vi "IMAQ FPGA FIFO to Pixel Bus RGB32x1.vi"(6 "Ready For Output":bool=TRUE, 10 "Image Size":T2, 11 "Source Image FIFO":refnum<k21>) -> (0 "Output Valid":bool, 2 "Source FIFO Status":T1, 3 "Pixel Bus Out":T3)   [LabVIEW 2017, in "NI_VDM_FPGA_Basics.lvlib"]
doc: "Reads image pixels out of the specified FIFO and returns a Pixel Bus cluster of the requested type. The Pixel Bus contains the pixel data from the FIFO along with some additional flags that indicate when the pixel data is valid, an end of a line has been reached, or an end of the image has been reached. The Pixel Bus is used to pass image data to all of the other VIs in the NI Vision Development Module for FPGA library. Only one of the DV, EOL, and EOI flags in the Pixel Bus cluster will assert on a given clock cycle. When the last pixel of an image is reached, the Pixel Bus will contain the pixel data and the DV flag will be TRUE and the EOL and EOI flags will be FALSE. The next clock cycle, the EOL flag will be TRUE and the DV and EOI flags will be FALSE. The following clock cycle, the EOI flag will be TRUE and the DV and EOL flags will be FALSE."
uses:
  <vilib>/visionFPGA/NI_VDM_FPGA_Basics.lvlib
  <vilib>/rvi/DataTransferAndStorage/Container/XNode/niFpgaContainer.xnode
  <vilib>/rvi/FIFO/Fifo_Resource/niFpgaFifoEmulationRefIn.vi
  <vilib>/visionFPGA/Controls/IMAQ FPGA Pixel Bus RGB32x1.ctl
  <vilib>/visionFPGA/Controls/IMAQ FPGA Source FIFO Status.ctl
  <vilib>/visionFPGA/Controls/IMAQ FPGA Image Size.ctl
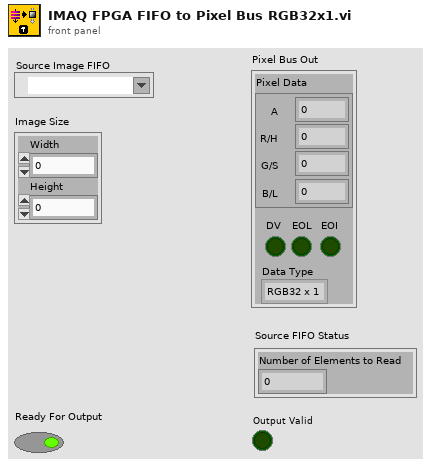
[diagram p1: front panel]
types:
  T1 = typedef "IMAQ FPGA Source FIFO Status.ctl" = cluster{"Number of Elements to Read":u32}
  T2 = typedef "IMAQ FPGA Image Size.ctl" = cluster{"Width":u32, "Height":u32}
  T3 = typedef "IMAQ FPGA Pixel Bus RGB32x1.ctl" = cluster{"Pixel Data":cluster{"A":u8, "R/H":u8, "G/S":u8, "B/L":u8}, "DV":bool, "EOL":bool, "EOI":bool, "Data Type":enum16{"RGB32 x 1"}}
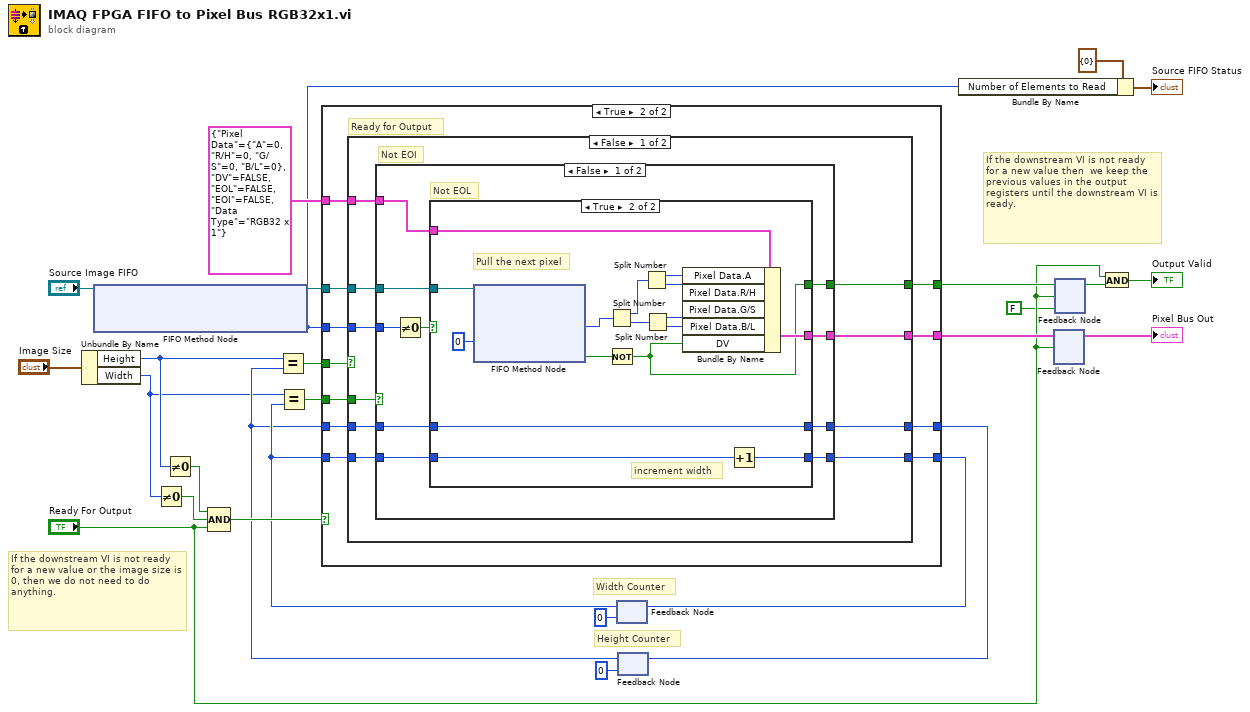
[diagram p0: block diagram]
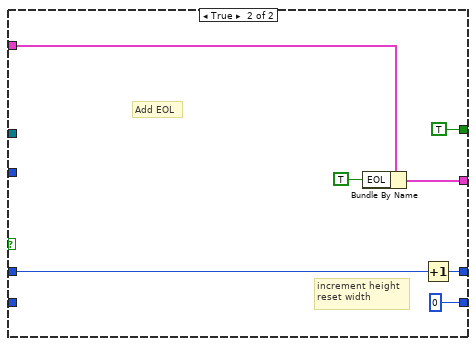
[diagram p4: hidden frame]
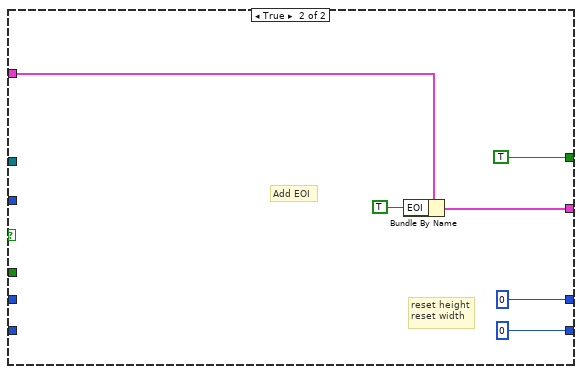
[diagram p5: hidden frame]
diagram:
  # "If the downstream VI is not ready for a new value or the image size is 0, then we do not need to do anything."
  # "If the downstream VI is not ready for a new value then  we keep the previous values in the output registers until the downstream VI is ready."
  # "Height Counter"
  # "Width Counter"
  n1 = Unbundle By Name("Image Size") -> ("Height"=w12:u32, "Width"=w11:u32)
  n2 = xnode ("FIFO Method Node")("FIFO In"="Source Image FIFO") -> ("Number of Elements to Read"=w1:u32, "FIFO Out"=w19:refnum<k21>)
  n3 = Not Equal To 0?(x=w11) -> (x != 0?=w17:bool)
  n4 = Not Equal To 0?(x=w12) -> (x != 0?=w16:bool)
  n5 = Compound Arithmetic op=AND(w16, w17, "Ready For Output") -> (w18:bool)
  n6 = feedback #1(u32 0 ("Image Width")) -> (w15:u32)
  n7 = Equal?(x=w11, y=w15) -> (x = y?=w25:bool)
  n8 = feedback #2(u32 0 ("Image Width")) -> (w14:u32)
  n9 = Equal?(x=w12, y=w14) -> (x = y?=w26:bool)
  n10 = case shown="True" w18 {
    tunnel: w26 -> [_ w40]
    tunnel: T3 {"Pixel Data"={"A"=0, "R/H"=0, "G/S"=0, "B/L"=0}, "DV"=FALSE, "EOL"=FALSE, "EOI"=FALSE, "Data Type"=enum."RGB32 x 1"} ("Pixel Bus Out") -> [_ w39]
    tunnel: w25 -> [_ w38]
    tunnel: w1 -> [_ w37]
    tunnel: [_ w36] -> w24
    tunnel: [w28 w35] -> w22
    tunnel: w15 -> [w28 w34]
    tunnel: [w29 w33] -> w20
    tunnel: w14 -> [w29 w32]
    tunnel: [_ w31] -> w10
    tunnel: w19 -> [_ w30]
    frame False {
      # "Do nothing...\nDown stream VI is not ready for new data."
    }
    frame True {
      # "Ready for Output"
      n11 = case shown="False" w40 {
        tunnel: w38 -> [w50 _]
        tunnel: [w49 TRUE ("EOI")] -> w36
        tunnel: [w48 w87] -> w31
        tunnel: w32 -> [w47 _]
        tunnel: w34 -> [w46 _]
        tunnel: [w45 u16 0 ("Height Counter")] -> w33
        tunnel: [w44 u16 0 ("Width Counter")] -> w35
        tunnel: w37 -> [w43 _]
        tunnel: w39 -> [w42 w86]
        tunnel: w30 -> [w41 _]
        frame False {
          # "Not EOI"
          n12 = case shown="False" w50 {
            tunnel: [w58 w84] -> w48
            tunnel: [w57 TRUE ("EOI")] -> w49
            tunnel: w47 -> [w56 w82]
            tunnel: w46 -> [w55 _]
            tunnel: [w53 w80] -> w45
            tunnel: [w54 u16 0 ("Width Counter")] -> w44
            tunnel: w43 -> [w59 _]
            tunnel: w42 -> [w52 w79]
            tunnel: w41 -> [w51 _]
            frame False {
              # "Not EOL"
              n13 = Not Equal To 0?(x=w59) -> (x != 0?=w60:bool)
              n14 = case shown="True" w60 {
                tunnel: [_ w77] -> w58
                tunnel: [_ w63] -> w57
                tunnel: w56 -> [w61 w74]
                tunnel: w55 -> [w62 w76]
                tunnel: [w62 w75] -> w54
                tunnel: [w61 w74] -> w53
                tunnel: w52 -> [_ w72]
                tunnel: w51 -> [_ w71]
                frame False {
                  # "Do nothing...\nnot EOI, not EOL, \nand no DMA data available"
                }
                frame True {
                  # "increment width"
                  # "Pull the next pixel"
                  n15 = xnode ("FIFO Method Node")("Timeout"=0, "FIFO In"=w71) -> ("Element"=w64:u32, "Timed Out?"=w73:bool)  [unwired: 1 out]
                  n16 = Split Number(x=w64) -> (hi(x)=w68:u16, lo(x)=w65:u16)
                  n17 = Not(x=w73) -> (.not. x?=w63:bool)
                  n18 = Split Number(x=w68) -> (hi(x)=w70:u8, lo(x)=w69:u8)
                  n19 = Split Number(x=w65) -> (hi(x)=w66:u8, lo(x)=w67:u8)
                  n20 = Bundle By Name(cluster=w72, "Pixel Data.A"=w70, "Pixel Data.R/H"=w69, "Pixel Data.G/S"=w66, "Pixel Data.B/L"=w67, "DV"=w63) -> (w77:T3)
                  n21 = Increment(x=w76) -> (x+1=w75:u32)
                }
              }
            }
            frame True {
              # "increment height\nreset width"
              # "Add EOL"
              n22 = Bundle By Name(cluster=w79, "EOL"=TRUE) -> (w84:T3)
              n23 = Increment(x=w82) -> (x+1=w80:u32)
            }
          }
        }
        frame True {
          # "reset height\nreset width"
          # "Add EOI"
          n24 = Bundle By Name(cluster=w86, "EOI"=TRUE) -> (w87:T3)
        }
      }
    }
  }
  n25 = feedback-in #1(w22) -> ()
  n26 = feedback-in #2(w20) -> ()
  n27 = Bundle By Name(cluster=T1 {"Number of Elements to Read"=0} ("FIFO Status"), "Number of Elements to Read"=w1) -> (→"Source FIFO Status":T1)
  n28 = feedback-in #3(w10, "Ready For Output") -> ()
  n29 = feedback #3() -> (→"Pixel Bus Out":T3)  [unwired: 1 in]
  n30 = feedback-in #4(w24, "Ready For Output") -> ()
  n31 = feedback #4(FALSE ("EOI")) -> (w6:bool)
  n32 = And(x="Ready For Output", y=w6) -> (x .and. y?=→"Output Valid":bool)
